vi "Uncover-V2.2.vi"(3 "index (col)":i32, 4 "index (row)":i32) -> ()   [LabVIEW 2014]
uses:
  BackMapGlobalV2.2.vi
  ShowMapGlobalV2.2.vi
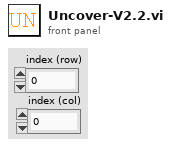
[diagram p1: front panel]
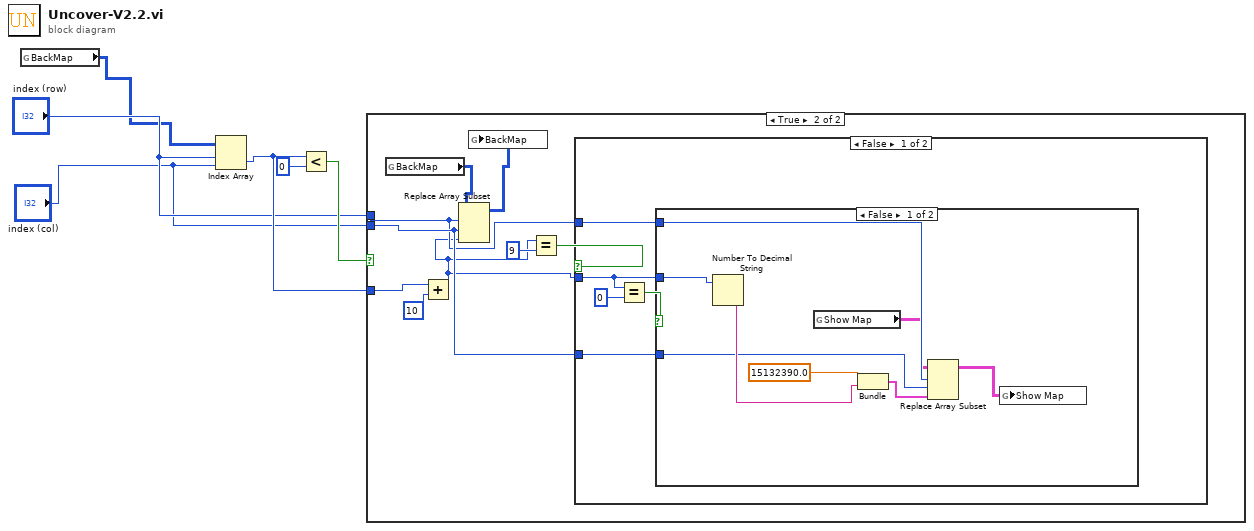
[diagram p0: block diagram]
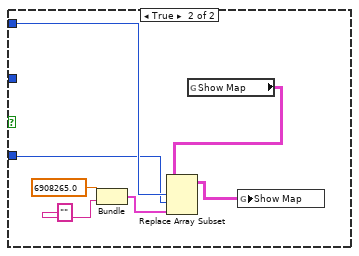
[diagram p3: hidden frame]
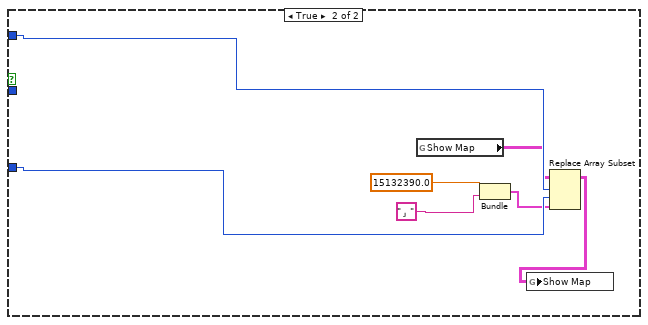
[diagram p4: hidden frame]
diagram:
  n1 = global read "BackMapGlobalV2.2.vi" "BackMap"() -> (w1:i32[][])
  n2 = Index Array(array=w1, index (row)="index (row)", index (col)="index (col)") -> (element=w4:i32)
  n3 = Less?(x=w4, y=0) -> (x < y?=w5:bool)
  n4 = case shown="True" w5 {
    tunnel: w4 -> [_ w15]
    tunnel: "index (row)" -> [_ w10]
    tunnel: "index (col)" -> [_ w11]
    frame False {
    }
    frame True {
      n5 = global read "BackMapGlobalV2.2.vi" "BackMap"() -> (w8:i32[][])
      n6 = Add(x=w15, y=10) -> (x+y=w9:i32)
      n7 = Replace Array Subset(array=w8, new element=w9, index (row)=w10, index (col)=w11) -> (w7:i32[][])
      n8 = global write "BackMapGlobalV2.2.vi" "BackMap"(w7) -> ()
      n9 = Equal?(x=w9, y=9) -> (x = y?=w12:bool)
      n10 = case shown="False" w12 {
        tunnel: w11 -> [w17 w41]
        tunnel: w10 -> [w18 w42]
        tunnel: w9 -> [w16 _]
        frame False {
          n11 = Equal?(x=w16, y=0) -> (x = y?=w19:bool)
          n12 = case shown="False" w19 {
            tunnel: w18 -> [w24 w32]
            tunnel: w17 -> [w23 w31]
            tunnel: w16 -> [w28 _]
            frame False {
              n13 = Number To Decimal String(number=w28) -> (decimal integer string=w25:string)  [unwired: 1 in]
              n14 = global read "ShowMapGlobalV2.2.vi" "Show Map"() -> (w22:cluster{"Color Box":u32, "String":string}[][])
              n15 = Bundle(15132390.0, w25) -> (w26:cluster{dbl, string})  [unwired: 1 in]
              n16 = Replace Array Subset(array=w22, new element=w26, index (row)=w24, index (col)=w23) -> (w21:cluster{"Color Box":u32, "String":string}[][])
              n17 = global write "ShowMapGlobalV2.2.vi" "Show Map"(w21) -> ()
            }
            frame True {
              n18 = Bundle(6908265.0, "") -> (w33:cluster{dbl, string})  [unwired: 1 in]
              n19 = global read "ShowMapGlobalV2.2.vi" "Show Map"() -> (w30:cluster{"Color Box":u32, "String":string}[][])
              n20 = Replace Array Subset(array=w30, new element=w33, index (row)=w32, index (col)=w31) -> (w29:cluster{"Color Box":u32, "String":string}[][])
              n21 = global write "ShowMapGlobalV2.2.vi" "Show Map"(w29) -> ()
            }
          }
        }
        frame True {
          n22 = global read "ShowMapGlobalV2.2.vi" "Show Map"() -> (w37:cluster{"Color Box":u32, "String":string}[][])
          n23 = Bundle(15132390.0, "」") -> (w38:cluster{dbl, string})  [unwired: 1 in]
          n24 = Replace Array Subset(array=w37, new element=w38, index (row)=w42, index (col)=w41) -> (w36:cluster{"Color Box":u32, "String":string}[][])
          n25 = global write "ShowMapGlobalV2.2.vi" "Show Map"(w36) -> ()
        }
      }
    }
  }
